vi "sent by stage QM.vi"(8 "error in (no error)":errorcluster, 10 "ProceedMessage":refnum<class "ProceedMessage.lvclass">, 11 "Thorcam in":refnum<class "Thorcam.lvclass">) -> (0 "error out":errorcluster, 2 "send by stage?":bool, 3 "Thorcam out":refnum<class "Thorcam.lvclass">)   [LabVIEW 2012, in "Thorcam.lvclass"]
uses:
  Thorcam.lvclass
  <vilib>/Distrio/Murmex/ProceedMessage/ProceedMessage.lvclass
  Thorcam.lvclass/Thorcam.ctl
  <vilib>/Distrio/Murmex/Message/Message.lvclass
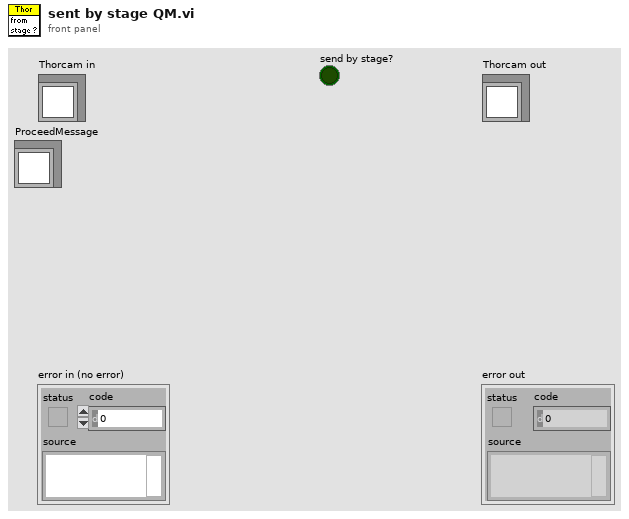
[diagram p1: front panel]
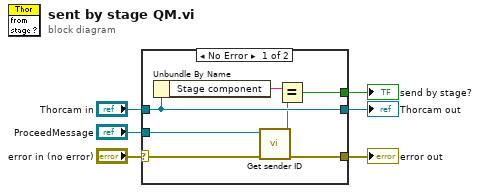
[diagram p0: block diagram]
diagram:
  n1 = case shown="No Error" "error in (no error)" {
    selector: "error in (no error)" -> [w13 w15]
    tunnel: [w11 w15] -> w5
    tunnel: [w12 w14] -> w3
    tunnel: "Thorcam in" -> [w12 w14]
    tunnel: "ProceedMessage" -> [w10 _]
    tunnel: [w7 _] -> w1
    frame No Error {
      n2 = Unbundle By Name(w12) -> ("Stage component"=w9:string)
      n3 = call <vilib>:"Get sender ID.vi"("error in (no error)"=w13, "Message in"=w10) -> ("error out"=w11:errorcluster, "sender"=w8:string)  [unwired: 7 in, 1 out]
      n4 = Equal?(x=w9, y=w8) -> (x = y?=w7:bool)
    }
    frame Error {
    }
  }
  "error out" <- w5
  "Thorcam out" <- w3
  "send by stage?" <- w1
